vi "Find Linearity Descriptors.vi"(8 "error in (no error)":errorcluster, 11 "Calibration Points":T1[](array[typedef])) -> (0 "error out":errorcluster, 3 "Linearity Fit Descriptors":T2(array[cluster]))   [LabVIEW 2026, in "Analysis.lvlib"]
uses:
  Analysis.lvlib
  controls/Messaging Payloads/Calibration Point Table Insert.ctl
  Linearity Descriptors.ctl
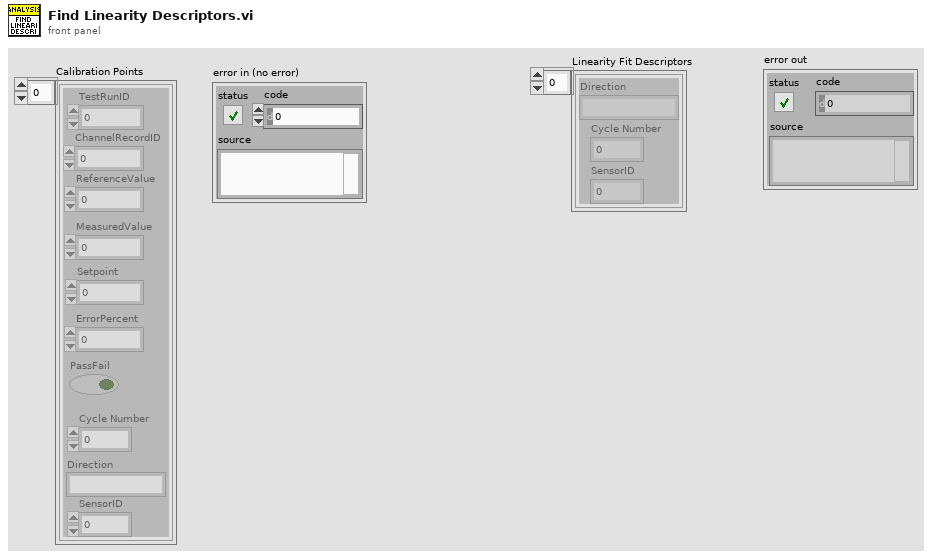
[diagram p1: front panel]
types:
  T1 = typedef "Calibration Point Table Insert.ctl" = cluster{"TestRunID":i32, "ChannelRecordID":i32, "Setpoint":dbl, "MeasuredValue":dbl, "ErrorPercent":dbl, "PassFail":bool, "ReferenceValue":dbl, "Cycle Number":i32, "Direction":string, "SensorID":i32}
  T2 = cluster{"Direction":string, "Cycle Number":i32, "SensorID":i32}[]
  T3 = typedef "Analysis.lvlib/Linearity Descriptors.ctl" = cluster{"Direction":string, "Cycle Number":i32, "SensorID":i32}
  T4 = cluster{"Direction":string, "Cycle Number":i32, "SensorID":i32}
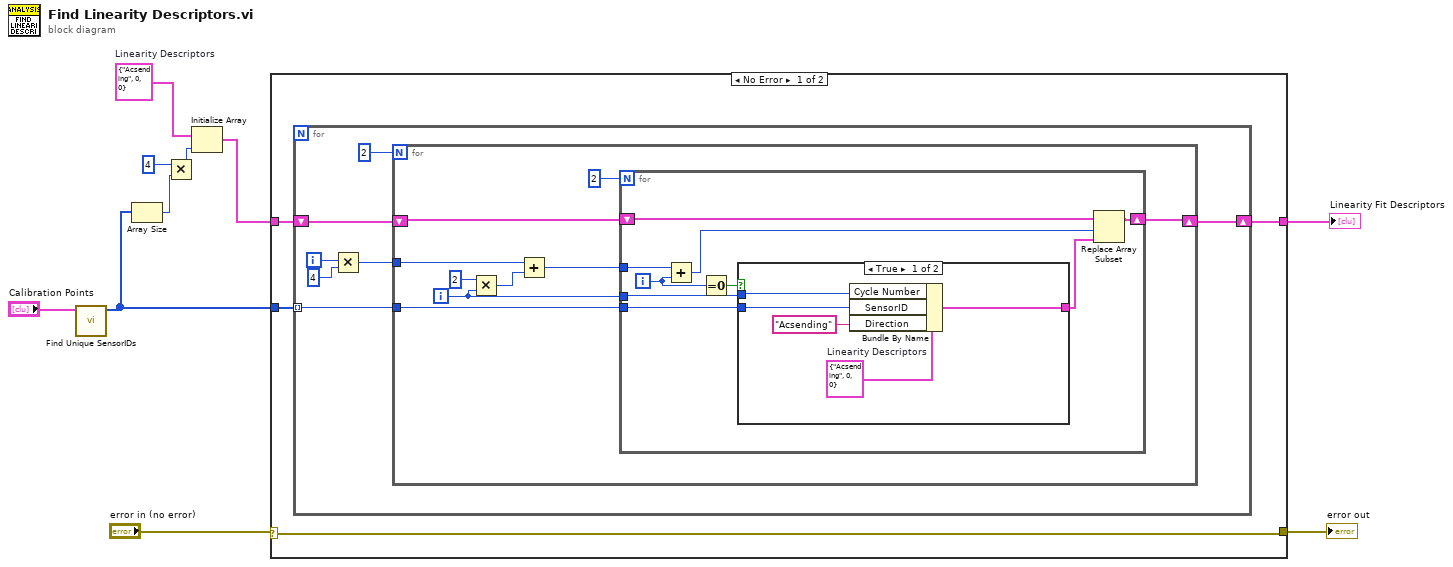
[diagram p0: block diagram]
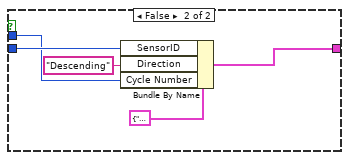
[diagram p2: hidden frame]
diagram:
  w7 = T3 {"Direction"="Acsending", "Cycle Number"=0, "SensorID"=0}  # Linearity Descriptors
  n1 = call "Find Unique SensorIDs.vi"("Calibration Points in"="Calibration Points") -> ("SensorIDs"=w6:i32[])  [unwired: 9 in, 1 out]
  n2 = Array Size(array=w6) -> (size(s)=w4:i32)
  n3 = Multiply(x=4, y=w4) -> (x*y=w5:i32)
  n4 = Initialize Array(w7, w5) -> (w8:T3[])
  n5 = case shown="No Error" "error in (no error)" {
    selector: "error in (no error)" -> [w11 w51]
    tunnel: [w14 w50] -> w10
    tunnel: w8 -> [w13 w50]
    tunnel: w6 -> [w12 _]
    tunnel: [w11 w51] -> w1
    frame No Error {
      n6 = for {
        tunnel: w12 -> [w21] mode=indexing
        shift-right: [w19] -> w14
        shift-left: w13 -> [w18]
        i -> [w16]
        n7 = Multiply(x=w16, y=4) -> (x*y=w15:i32)
        n8 = for {
          N: 2 -> [_]
          tunnel: w21 -> [w30]
          shift-right: [w28] -> w19
          shift-left: w18 -> [w29]
          tunnel: w15 -> [w27]
          i -> [w22]
          n9 = Multiply(x=2 ("y"), y=w22) -> (x*y=w26:i32)
          n10 = Add(x=w27, y=w26) -> (x+y=w25:i32)
          n11 = for {
            N: 2 -> [_]
            tunnel: w22 -> [w39]
            tunnel: w30 -> [w38]
            shift-right: [w34] -> w28
            shift-left: w29 -> [w35]
            tunnel: w25 -> [w33]
            i -> [w31]
            n12 = Add(x=w33, y=w31) -> (x+y=w32:i32)
            n13 = Equal To 0?(x=w31) -> (x = 0?=w37:bool)
            n14 = case shown="True" w37 {
              tunnel: w39 -> [w41 w45]
              tunnel: w38 -> [w43 w47]
              tunnel: [w44 w49] -> w36
              frame True {
                w40 = T3 {"Direction"="Acsending", "Cycle Number"=0, "SensorID"=0}  # Linearity Descriptors
                n15 = Bundle By Name(cluster=w40, "Cycle Number"=w41, "SensorID"=w43, "Direction"="Acsending") -> (w44:T3)
              }
              frame False {
                n16 = Bundle By Name(cluster=T4 {"Direction"="Acsending", "Cycle Number"=0, "SensorID"=0} ("input cluster"), "SensorID"=w47, "Direction"="Descending", "Cycle Number"=w45) -> (w49:T4)
              }
            }
            n17 = Replace Array Subset(array=w35, new element=w36, index=w32) -> (w34:T3[])
          }
        }
      }
    }
    frame Error {
    }
  }
  "Linearity Fit Descriptors" <- w10
  "error out" <- w1
